vi "Receive Control Key Down Event.vi"(8 "error in (no error)":errorcluster, 10 "ControlKeyDownMsg":refnum<class "ControlKeyDownMsg.lvclass">, 11 "Login View In":refnum<class "Login View.lvclass">) -> (0 "error out":errorcluster, 3 "Login View Out":refnum<class "Login View.lvclass">)   [LabVIEW 2017, in "Login View.lvlib" / "Login View.lvclass"]
doc: "<License>\nCopyright © 2017 Composed Systems, LLC | All rights reserved\nwww.composed.io\n\nAuthor: Ethan Stern <ethan.stern@composed.io>\n\nThis software is provided \"AS IS\" WITHOUT WARRANTIES, either express or implied, AND IS FOR EDUCATIONAL PURPOSES ONLY.\n</License>"
uses:
  Login View.lvclass
  <vilib>/gpm_packages/@cs/mva-viewable/Source/ActorEvents/IEventAggregator Messages/ControlKeyDownMsg/ControlKeyDownMsg.lvclass
  <vilib>/gpm_packages/@cs/mva-viewable/Source/ActorEvents/IEventAggregator Messages/ControlKeyDownMsg/ControlKeyDownMsg.lvclass/ControlKeyDownMsg.ctl
  Login View.lvclass/Login View.ctl
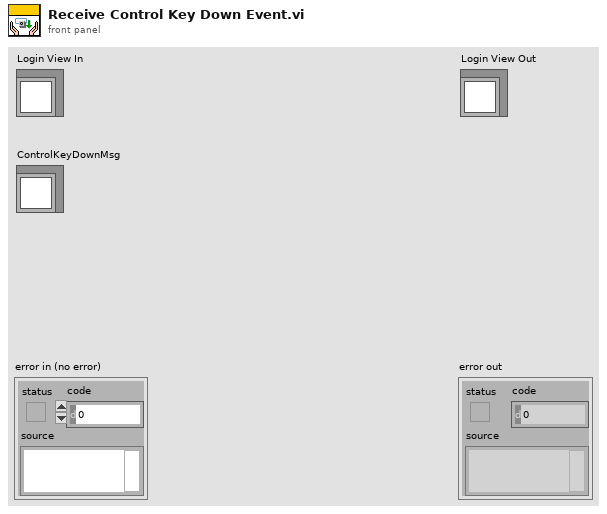
[diagram p1: front panel]
types:
  T1 = typedef "eventvkey.ctl" = enum16{"ASCII", "Enter", "Return", "Shift", "Ctrl", "Alt", "Cmd", "Opt", "Caps", "NumLock", "Clear", "Break", "Up", "Down", "Left", "Right", "Insert", "Delete", "Home", "End", "PageUp", "PageDown", "Escape", "Help", "Pause", "ScrollLock", "F1", "F2", "F3", "F4", "F5", "F6", "F7", "F8", "F9", "F10", "F11", "F12", "F13", "F14", "F15", "F16", "F17", "F18", "F19", "F20", "F21", "F22", "F23", "F24", "Play", "VolumeUp", "VolumeDown", "Mute", "Two Byte Char"}
  T2 = typedef "User Manager Application Types.lvlib/Credentials.ctl" = cluster{"Username":string, "Password":string}
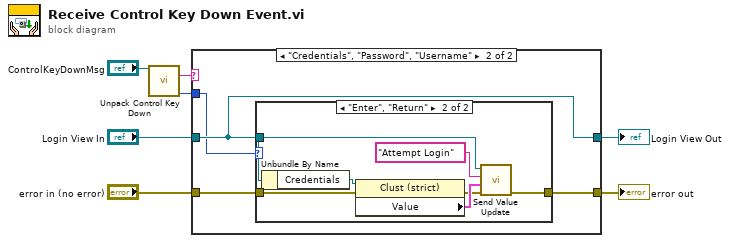
[diagram p0: block diagram]
diagram:
  n1 = call <vilib>:"Unpack Control Key Down.vi"("ControlKeyDownMsg"="ControlKeyDownMsg") -> ("Control Label"=w6:string, "VKey"=w1:T1)  [unwired: 6 in, 7 out]
  n2 = case shown="\"Credentials\", \"Password\", \"Username\"" w6 {
    tunnel: [w8 w10] -> w3
    tunnel: [w9 w13] -> w4
    tunnel: "error in (no error)" -> [w8 w12]
    tunnel: "Login View In" -> [w9 w13]
    tunnel: w1 -> [_ w11]
    frame "False", Default {
    }
    frame "Credentials", "Password", "Username" {
      n3 = case shown="\"Enter\", \"Return\"" w11 {
        tunnel: [w14 w21] -> w10
        tunnel: w13 -> [_ w19]
        tunnel: w12 -> [w14 w15]
        frame Default {
        }
        frame "Enter", "Return" {
          n4 = Unbundle By Name(w19) -> ("Credentials"=w18:refnum<vi>)
          n5 = property class="Clust (strict)"(reference=w18, error in=w15) -> (error out=w16:errorcluster, "Value"=w17:T2)  [unwired: 1 out]
          n6 = call-dynamic "Send Value Update.vi"("error in (no error)"=w16, "Value"=w17, "Datum Name"="Attempt Login", "IViewable in"=w19) -> ("error out"=w21:errorcluster)  [unwired: 7 in]
        }
      }
    }
  }
  "error out" <- w3
  "Login View Out" <- w4
